vi "Omni-teste-slow.vi"() -> ()   [LabVIEW 2012]
panel:
  out "time":u32
  in  "stop":bool
  out "XY Graph":T1(graph)
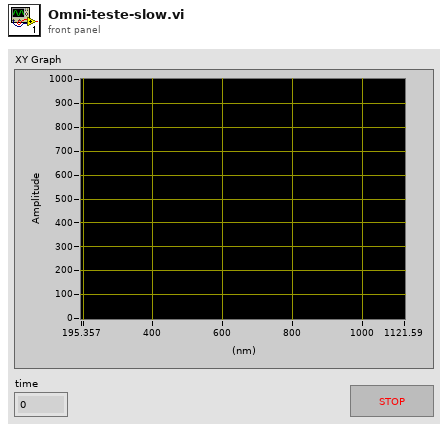
[diagram p1: front panel]
types:
  T1 = cluster{"WL Values":dbl[], "Spectrum Values":dbl[]}
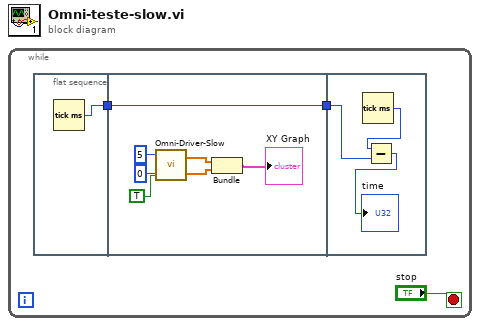
[diagram p0: block diagram]
diagram:
  n1 = while {
    stop <- "stop" stop-if-true
    n2 = flat-sequence {
      tunnel: [w4] -> w2
      tunnel: w2 -> [w5]
      tunnel: [w5] -> w1
      tunnel: w1 -> [w13]
      frame #0 {
        n3 = Tick Count (ms)() -> (millisecond timer value=w4:u32)
      }
      frame #1 {
        n4 = call "Omni-Driver-Slow.vi"("Correct Electrical Dark"=TRUE, "Spectrometer number"=0, "Integration Time (ms)"=5) -> ("Spectrum Values"=w10:dbl[], "WL Values"=w11:dbl[])
        n5 = Bundle("WL Values"=w11, "Spectrum Values"=w10) -> (→"XY Graph":T1)  [unwired: 1 in]
      }
      frame #2 {
        n6 = Tick Count (ms)() -> (millisecond timer value=w14:u32)
        n7 = Subtract(x=w14, y=w13) -> (x-y=→"time":u32)
      }
    }
  }
